vi "WS1050_AD7747_VSA_Cap Bank Setting.vi"(0 "Select Com Port":refnum<visa-resource-name>="COM8", 3 "Push Button to write Offset":bool, 5 "errorin":errorcluster, 6 "Click down to quit":bool, 7 "Push Button to Measue Cap":bool=TRUE, 9 "CApDac_values":string[](array[string])=["900bA5", "900bA4", "900bA5"], 10 "Push Button to Initialize AD7747":bool, 12 "Push Button to Calibrate":bool) -> (11 "C3_Meas(pF)":string, 13 "Com Port Out":refnum<visa-resource-name>="COM1", 14 "C2(pF)":dbl, 15 "C1_Meas(pF)":string, 16 "C2_Meas(pF)":string, 17 "C1(pF)":dbl, 18 "C3(pF)":dbl, 19 "error out":errorcluster)   [LabVIEW 2012]
panel:
  # "AD7747 Control Ver1.0"
  # "Interface PIC I2C Control"
  # "Bank Cap Measurements"
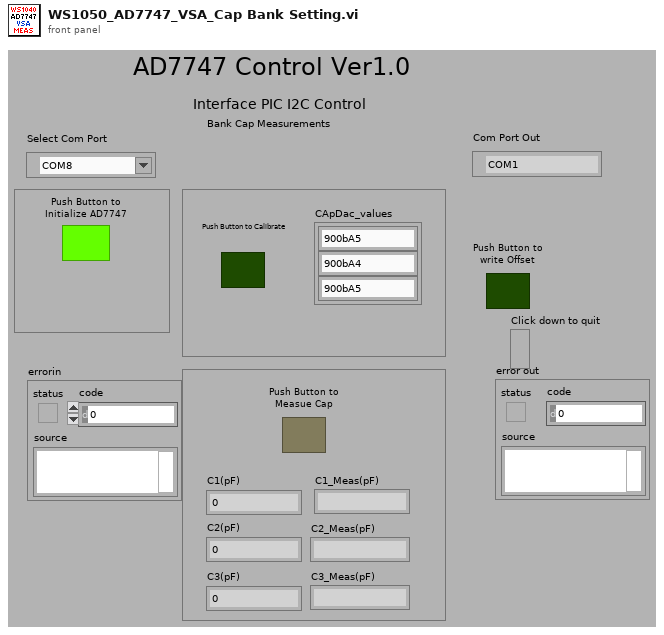
[diagram p1: front panel]
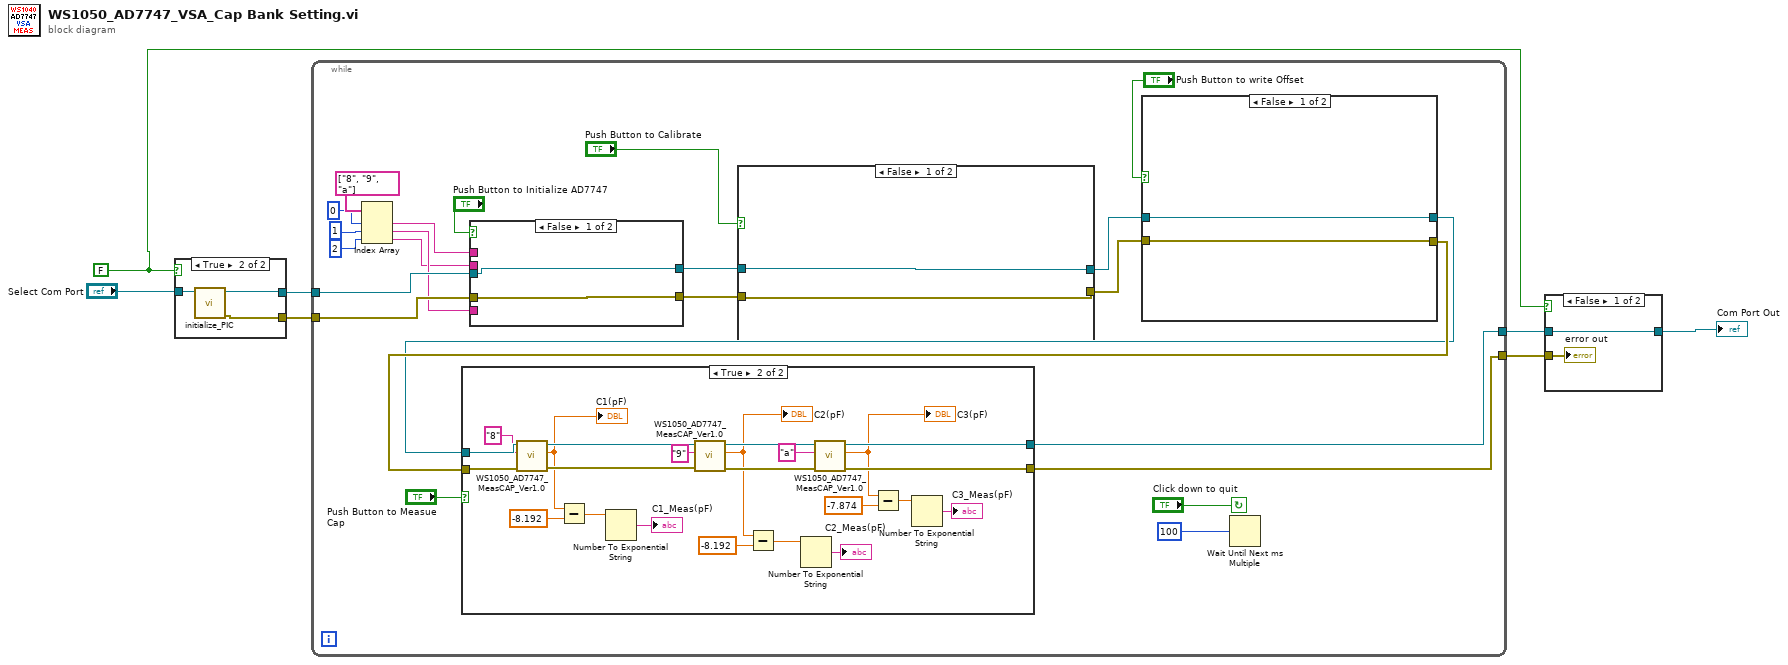
[diagram p0: block diagram]
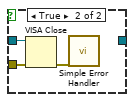
[diagram p2: hidden frame]
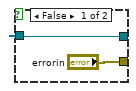
[diagram p3: hidden frame]
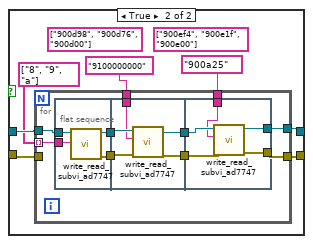
[diagram p4: hidden frame]
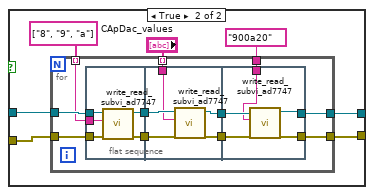
[diagram p5: hidden frame]
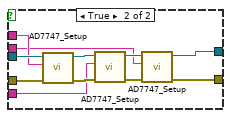
[diagram p6: hidden frame]
diagram:
  w2 = FALSE
  n1 = case shown="True" w2 {
    tunnel: ["errorin" w12] -> w7
    tunnel: [w8 w11] -> w6
    tunnel: "Select Com Port" -> [w8 w10]
    frame False {
    }
    frame True {
      n2 = call "initialize_PIC.vi"("Select Com Port"=w10) -> ("error out"=w12:errorcluster, "VISA resource name out"=w11:refnum<visa-resource-name>)  [unwired: 9 in]
    }
  }
  n3 = while {
    tunnel: w7 -> [w30]
    tunnel: w6 -> [w28]
    tunnel: [w17] -> w5
    tunnel: [w35] -> w4
    stop <- "Click down to quit" continue-if-true
    n4 = Index Array(array=string[] ["8", "9", "a"], index #1=0 ("index"), index #2=1 ("index"), index #3=2 ("index")) -> (element #1=w31:string, element #2=w24:string, element #3=w23:string)
    n5 = case shown="False" "Push Button to Initialize AD7747" {
      tunnel: w30 -> [w104 w115]
      tunnel: [w104 w105] -> w18
      tunnel: w28 -> [w103 w114]
      tunnel: w31 -> [_ w109]
      tunnel: w24 -> [_ w108]
      tunnel: w23 -> [_ w107]
      tunnel: [w103 w106] -> w15
      frame False {
      }
      frame True {
        n6 = call "AD7747_Setup.vi"("error in"=w115, "AD7747_Number"=w109, "Control"=w114) -> ("error out"=w113:errorcluster, "Control out"=w112:refnum<visa-resource-name>)  [unwired: 6 in, 1 out]
        n7 = call "AD7747_Setup.vi"("error in"=w113, "AD7747_Number"=w108, "Control"=w112) -> ("error out"=w111:errorcluster, "Control out"=w110:refnum<visa-resource-name>)  [unwired: 6 in, 1 out]
        n8 = call "AD7747_Setup.vi"("error in"=w111, "AD7747_Number"=w107, "Control"=w110) -> ("error out"=w105:errorcluster, "Control out"=w106:refnum<visa-resource-name>)  [unwired: 6 in, 1 out]
      }
    }
    n9 = case shown="False" "Push Button to Calibrate" {
      tunnel: [w69 w77] -> w29
      tunnel: w18 -> [w69 w74]
      tunnel: w15 -> [w70 w73]
      tunnel: [w70 w72] -> w14
      frame False {
      }
      frame True {
        n10 = for {
          tunnel: [w83] -> w77
          tunnel: w73 -> [w87]
          tunnel: w74 -> [w88]
          tunnel: string[] ["8", "9", "a"] -> [w86] mode=indexing
          tunnel: "CApDac_values" -> [w82] mode=indexing
          tunnel: [w81] -> w72
          tunnel: "900a20" ("Data_In 2") -> [w78]
          n11 = flat-sequence {
            tunnel: w88 -> [w93]
            tunnel: w87 -> [w91]
            tunnel: w86 -> [w89]
            tunnel: [w92] -> w85
            tunnel: [w90] -> w84
            tunnel: w85 -> [w97]
            tunnel: w84 -> [w98]
            tunnel: w82 -> [w95]
            tunnel: [w96] -> w80
            tunnel: [w94] -> w79
            tunnel: [w100] -> w81
            tunnel: [w102] -> w83
            tunnel: w80 -> [w102]
            tunnel: w79 -> [w101]
            tunnel: w78 -> [w99]
            frame #0 {
              n12 = call "write_read_subvi_ad7747.vi"("error in (no error)"=w93, "command"=w89, "Control"=w91) -> ("error out"=w92:errorcluster, "Control out"=w90:refnum<visa-resource-name>)  [unwired: 6 in, 1 out]
            }
            frame #1 {
              n13 = call "write_read_subvi_ad7747.vi"("error in (no error)"=w97, "command"=w95, "Control"=w98) -> ("error out"=w96:errorcluster, "Control out"=w94:refnum<visa-resource-name>)  [unwired: 6 in, 1 out]
            }
            frame #2 {
              n14 = call "write_read_subvi_ad7747.vi"("command"=w99, "Control"=w101) -> ("Control out"=w100:refnum<visa-resource-name>)  [unwired: 7 in, 2 out]
            }
          }
        }
      }
    }
    n15 = case shown="False" "Push Button to write Offset" {
      tunnel: w14 -> [w36 w43]
      tunnel: w29 -> [w37 w44]
      tunnel: [w37 w41] -> w16
      tunnel: [w36 w40] -> w13
      frame False {
      }
      frame True {
        (unwired) string[] ["900ef4", "900e1f", "900e00"]
        (unwired) string[] ["900d98", "900d76", "900d00"]
        n16 = for {
          tunnel: w44 -> [_]
          tunnel: [w48] -> w41
          tunnel: w43 -> [w54]
          tunnel: string[] ["8", "9", "a"] -> [w53] mode=indexing
          tunnel: "9100000000" ("Data_In 2") -> [w47]
          tunnel: "900a25" ("Data_In 2") -> [w46]
          tunnel: [w45] -> w40
          n17 = flat-sequence {
            tunnel: w54 -> [w56]
            tunnel: w53 -> [w55]
            tunnel: [w58] -> w52
            tunnel: [w57] -> w51
            tunnel: w52 -> [w61]
            tunnel: w51 -> [w63]
            tunnel: [w60] -> w50
            tunnel: [w62] -> w49
            tunnel: w47 -> [w59]
            tunnel: w50 -> [w67]
            tunnel: w49 -> [w68]
            tunnel: [w66] -> w48
            tunnel: w46 -> [w65]
            tunnel: [w64] -> w45
            frame #0 {
              n18 = call "write_read_subvi_ad7747.vi"("command"=w55, "Control"=w56) -> ("error out"=w58:errorcluster, "Control out"=w57:refnum<visa-resource-name>)  [unwired: 7 in, 1 out]
            }
            frame #1 {
              n19 = call "write_read_subvi_ad7747.vi"("error in (no error)"=w61, "command"=w59, "Control"=w63) -> ("error out"=w60:errorcluster, "Control out"=w62:refnum<visa-resource-name>)  [unwired: 6 in, 1 out]
            }
            frame #2 {
              n20 = call "write_read_subvi_ad7747.vi"("error in (no error)"=w67, "command"=w65, "Control"=w68) -> ("error out"=w66:errorcluster, "Control out"=w64:refnum<visa-resource-name>)  [unwired: 6 in, 1 out]
            }
          }
        }
      }
    }
    n21 = case shown="True" "Push Button to Measue Cap" {
      tunnel: w16 -> [w117 w140]
      tunnel: w13 -> [w116 w139]
      tunnel: [w117 w131] -> w17
      tunnel: [w116 w130] -> w35
      frame False {
      }
      frame True {
        n22 = call "WS1050_AD7747_MeasCAP_Ver1.0.vi"("error in (no error)"=w140, "AD7747_Number"="8", "Control"=w139) -> ("error"=w136:errorcluster, "CAP (pF)"=w129:dbl, "Control out"=w135:refnum<visa-resource-name>)  [unwired: 5 in, 1 out]
        "C1(pF)" <- w129
        n23 = Subtract(x=w129, y=-8.192) -> (x-y=w119:dbl)
        n24 = Number To Exponential String(number=w119) -> (E-format string=→"C1_Meas(pF)":string)  [unwired: 3 in]
        n25 = call "WS1050_AD7747_MeasCAP_Ver1.0.vi"("error in (no error)"=w136, "AD7747_Number"="9", "Control"=w135) -> ("error"=w133:errorcluster, "CAP (pF)"=w128:dbl, "Control out"=w132:refnum<visa-resource-name>)  [unwired: 5 in, 1 out]
        "C2(pF)" <- w128
        n26 = Subtract(x=w128, y=-8.192) -> (x-y=w122:dbl)
        n27 = Number To Exponential String(number=w122) -> (E-format string=→"C2_Meas(pF)":string)  [unwired: 3 in]
        n28 = call "WS1050_AD7747_MeasCAP_Ver1.0.vi"("error in (no error)"=w133, "AD7747_Number"="a", "Control"=w132) -> ("error"=w131:errorcluster, "CAP (pF)"=w126:dbl, "Control out"=w130:refnum<visa-resource-name>)  [unwired: 5 in, 1 out]
        "C3(pF)" <- w126
        n29 = Subtract(x=w126, y=-7.874) -> (x-y=w124:dbl)
        n30 = Number To Exponential String(number=w124) -> (E-format string=→"C3_Meas(pF)":string)  [unwired: 3 in]
      }
    }
    n31 = Wait Until Next ms Multiple(millisecond multiple=u32 100) -> ()  [unwired: 1 out]
  }
  n32 = case shown="False" w2 {
    tunnel: w5 -> [w142 w144]
    tunnel: w4 -> [w141 w143]
    tunnel: [w141 _] -> w1
    frame False {
      "error out" <- w142
    }
    frame True {
      n33 = VISA Close(VISA resource name=w143, error in (no error)=w144) -> (error out=w145:errorcluster)
      n34 = call <vilib>:"Simple Error Handler.vi"("error in (no error)"=w145) -> ()  [unwired: 1 in, 8 out]
    }
  }
  "Com Port Out" <- w1
